vi "Configure Display.vi"(0 "VISA resource name":refnum<visa-resource-name>, 1 "Number of Custom\nDisplay Locations (0:2 Large)":u16(ring) items=["2 Large", "4 Large", "8 Small"], 2 "Bottom Half\nDisplayed Output (1:Output)":u16(ring)=1 items=["Output 1"=1, "Output 2"=2, "Output 3"=3, "Output 4"=4], 5 "Display Mode (0:Input A)":u16(ring) items=["Input A", "Input B", "Input C", "Input D", "Custom", "Four Loop"], 7 "Front Panel LEDs (T: On)":bool=TRUE, 9 "Contrast (28)":dbl=28.0, 11 "error in (no error)":errorcluster, 12 "Field to Configure (1)":dbl=1.0, 13 "Input (0:None)":u16(ring) items=["None", "Input A", "Input B", "Input C", "Input D"], 14 "Units (1:Kelvin)":u16(ring)=1 items=["Kelvin"=1, "Celsius"=2, "Sensor Units"=3, "Minimum Data"=4, "Maximum Data"=5]) -> (4 "VISA resource name out":refnum<visa-resource-name>, 15 "error out":errorcluster)   [LabVIEW 2019, in "Lake Shore 336.lvlib"]
doc: "This VI configures the Model 336 front panel display settings. The Model 336 provides several display modes designed to accommodate different instrument configurations and user preferences. The Four Loop diaplay mode offers large format sensor readings of each of the 4 sensor inputs as well as setpoint and heater output information for associated outputs, all on 1 screen. The Input display modes provide detailed information about the relevant sensor input, and the associated output. The Custom display mode provides a means for users to assign differeent types of information to specific sections of the display."
uses:
  Lake Shore 336.lvlib
  Instance           1 25Saved   Configure Display .vi
panel:
  # "Custom Display Mode Settings"
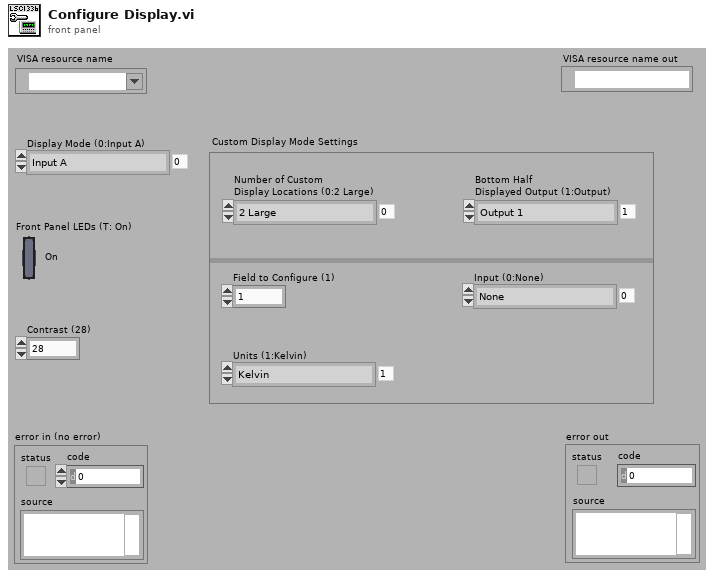
[diagram p1: front panel]
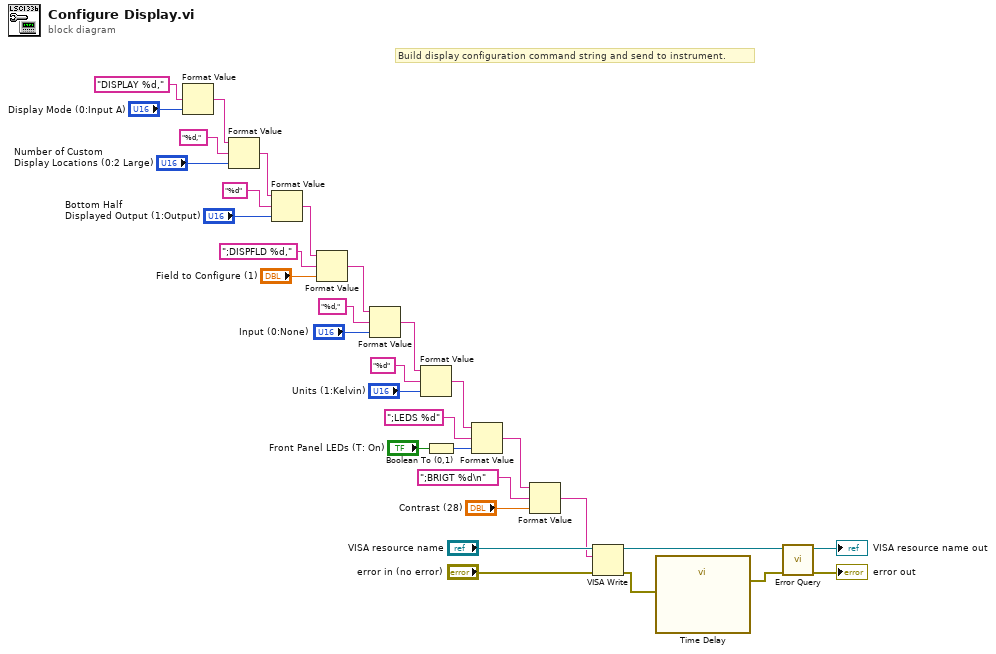
[diagram p0: block diagram]
diagram:
  # "Build display configuration command string and send to instrument."
  n1 = Format Value(format string="DISPLAY %d,", value (0)="Display Mode (0:Input A)") -> (output string=w13:string)  [unwired: 1 in]
  n2 = Format Value(string ("")=w13, format string="%d,", value (0)="Number of Custom\nDisplay Locations (0:2 Large)") -> (output string=w12:string)
  n3 = Format Value(string ("")=w12, format string="%d", value (0)="Bottom Half\nDisplayed Output (1:Output)") -> (output string=w9:string)
  n4 = Format Value(string ("")=w9, format string=";DISPFLD %d,", value (0)="Field to Configure (1)") -> (output string=w23:string)
  n5 = Format Value(string ("")=w23, format string="%d,", value (0)="Input (0:None)") -> (output string=w21:string)
  n6 = Format Value(string ("")=w21, format string="%d", value (0)="Units (1:Kelvin)") -> (output string=w5:string)
  n7 = Boolean To (0,1)(Boolean="Front Panel LEDs (T: On)") -> (0, 1=w8:i16)
  n8 = Format Value(string ("")=w5, format string=";LEDS %d", value (0)=w8) -> (output string=w3:string)
  n9 = Format Value(string ("")=w3, format string=";BRIGT %d\n", value (0)="Contrast (28)") -> (output string=w1:string)
  n10 = VISA Write(VISA resource name="VISA resource name", write buffer=w1, error in (no error)="error in (no error)") -> (VISA resource name out=w29:refnum<visa-resource-name>, error out=w19:errorcluster)  [unwired: 1 out]
  n11 = call "Time Delay"("error in (no error)"=w19) -> ("error out"=w18:errorcluster)  [unwired: 10 in]
  n12 = call "Error Query.vi"("error in (no error)"=w18, "VISA resource name"=w29) -> ("error out"=→"error out":errorcluster, "VISA resource name out"=→"VISA resource name out":refnum<visa-resource-name>)  [unwired: 7 in, 1 out]
